vi "User Get All.vi"(6 "Descending? (F)":bool, 8 "error in (no error)":errorcluster, 10 "Sort by Field (sxUsername)":T1, 11 "Connection Refnum":T2) -> (0 "error out":errorcluster, 2 "User Records":T3[](array[typedef]), 3 "Connection Refnum":T2, 4 "Data Present?":bool)   [LabVIEW 2011]
uses:
  User Record.ctl
  Summitek EXT/ODBC/SQL Controls/Connection Refnum.ctl
  User Record Fields.ctl
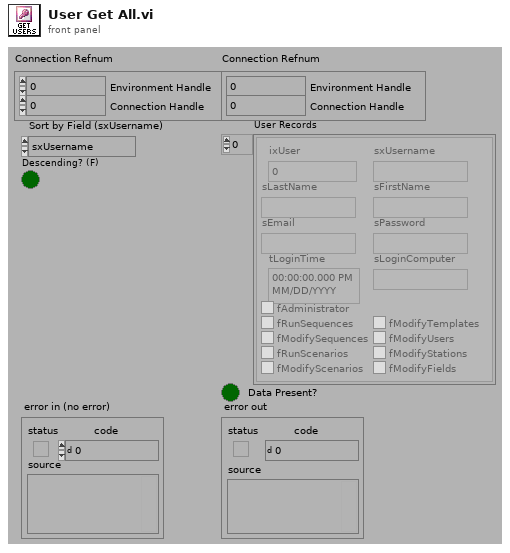
[diagram p1: front panel]
types:
  T1 = typedef "User Record Fields.ctl" = enum32{"sxUsername", "sLastName", "sFirstName", "sEmail", "sPassword", "tLoginTime", "sLoginComputer", "fAdministrator", "fRunSequences", "fModifySequences", "fRunScenarios", "fModifyScenarios", "fModifyTemplates", "fModifyUsers", "fModifyStations", "fModifyFields", "ixUser"}
  T2 = typedef "Connection Refnum.ctl" = cluster{"Environment Handle":i32, "Connection Handle":i32}
  T3 = typedef "User Record.ctl" = cluster{"ixUser":i32, "sxUsername":string, "sLastName":string, "sFirstName":string, "sEmail":string, "sPassword":string, "tLoginTime":timestamp, "sLoginComputer":string, "fAdministrator":bool, "fRunSequences":bool, "fModifySequences":bool, "fRunScenarios":bool, "fModifyScenarios":bool, "fModifyTemplates":bool, "fModifyUsers":bool, "fModifyStations":bool, "fModifyFields":bool}
  T4 = typedef "Statement Refnum.ctl" = cluster{"Statement Handle":i32, "Parameter Number":u16}
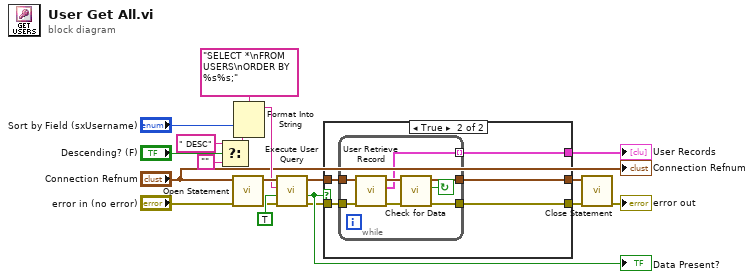
[diagram p0: block diagram]
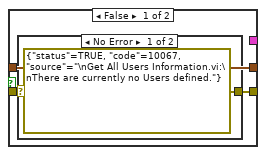
[diagram p2: hidden frame]
diagram:
  n1 = Select(t=" DESC" ("input 2"), s="Descending? (F)", f="") -> (s? t:f=w6:string)
  n2 = call "Open Statement.vi"("error in (no error)"="error in (no error)", "Connection Refnum"="Connection Refnum") -> ("error out"=w14:errorcluster, "Statement Refnum"=w15:T4)  [unwired: 4 out]
  n3 = Format Into String(format string="SELECT *\nFROM USERS\nORDER BY %s%s;" ("Query Name"), "Sort by Field (sxUsername)", w6) -> (resulting string=w11:string)  [unwired: 2 in, 1 out]
  n4 = call "Execute User Query.vi"("error in (no error)"=w14, "Return Data? (f)"=TRUE, "User Query"=w11, "Statement Refnum"=w15) -> ("error out"=w18:errorcluster, "Data Present?"=w19:bool, "Statement Refnum"=w17:T4)  [unwired: 1 out]
  "Data Present?" <- w19
  n5 = case shown="True" w19 {
    tunnel: w18 -> [w20 w29]
    tunnel: w17 -> [w22 w28]
    tunnel: [w21 w27] -> w13
    tunnel: [w22 w26] -> w12
    tunnel: [_ w25] -> w3
    frame False {
      n6 = case shown="No Error" w20 {
        selector: w20 -> [_ w24]
        tunnel: [errorcluster {"status"=TRUE, "code"=10067, "source"="\nGet All Users Information.vi:\nThere are currently no Users defined."} ("error out") w24] -> w21
        frame No Error {
        }
        frame Error {
        }
      }
    }
    frame True {
      n7 = while {
        tunnel: w29 -> [w36]
        tunnel: w28 -> [w31]
        tunnel: [w34] -> w27
        tunnel: [w33] -> w26
        tunnel: [w30] -> w25 mode=indexing
        stop <- w37 continue-if-true
        n8 = call "User Retrieve Record.vi"("error in (no error)"=w36, "Statement Refnum"=w31) -> ("error out"=w35:errorcluster, "User Record"=w30:T3, "Statement Refnum"=w32:T4)  [unwired: 7 out]
        n9 = call "Check for Data.vi"("error in (no error)"=w35, "Statement Refnum"=w32) -> ("error out"=w34:errorcluster, "Data Present?"=w37:bool, "Statement Refnum"=w33:T4)  [unwired: 3 out]
      }
    }
  }
  "User Records" <- w3
  n10 = call "Close Statement.vi"("error in (no error)"=w13, "Statement Refnum"=w12) -> ("error out"=→"error out":errorcluster)  [unwired: 5 out]
  "Connection Refnum" <- "Connection Refnum"
